vi "BuildPacketJ1939.vi"(7 "Priority":u8=6 format="%x", 9 "SA":u8, 10 "Data":u8[](array[numeric]), 11 "TxID":u8) -> (2 "MsgTX 2":T1)   [LabVIEW 2017]
panel:
  out "PGN":u16
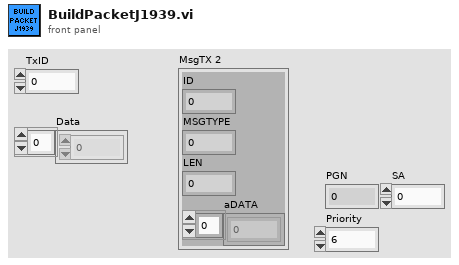
[diagram p1: front panel]
types:
  T1 = cluster{"ID":u32, "MSGTYPE":u8, "LEN":u8, "aDATA":u8[]}
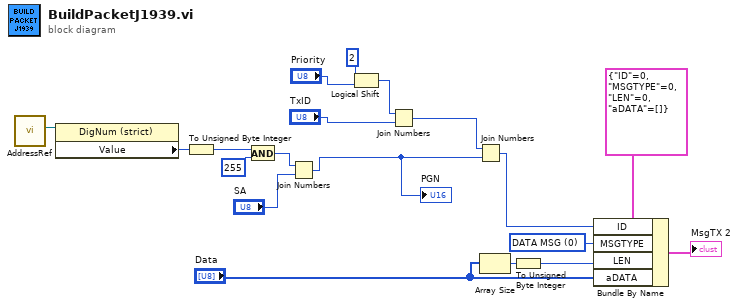
[diagram p0: block diagram]
diagram:
  w19 = u8 0 items=["STATUS"=128, "EXTENDED"=2, "RTR"=1, "DATA MSG"=0] ("MSGTYPE")
  n1 = call "AddressRef.vi"() -> ("add_type out"=w14:refnum<vi>)  [unwired: 9 in, 2 out]
  n2 = property class="DigNum (strict)"(reference=w14) -> ("Value"=w7:u16)  [unwired: 1 in, 2 out]
  n3 = To Unsigned Byte Integer(number=w7) -> (unsigned 8bit integer=w4:u8)
  n4 = And(x=w4, y=u8 255) -> (x .and. y?=w3:u8)
  n5 = Join Numbers(hi=w3, lo="SA") -> ((hi.lo)=w5:u16)
  "PGN" <- w5
  n6 = Logical Shift(y=i16 2, x="Priority") -> (x << y=w11:u8)
  n7 = Join Numbers(hi=w11, lo="TxID") -> ((hi.lo)=w8:u16)
  n8 = Join Numbers(hi=w8, lo=w5) -> ((hi.lo)=w13:u32)
  n9 = Array Size(array="Data") -> (size(s)=w15:i32)
  n10 = To Unsigned Byte Integer(number=w15) -> (unsigned 8bit integer=w18:u8)
  n11 = Bundle By Name(cluster=T1 {"ID"=0, "MSGTYPE"=0, "LEN"=0, "aDATA"=[]} ("MsgTX 2"), "ID"=w13, "MSGTYPE"=w19, "LEN"=w18, "aDATA"="Data") -> (→"MsgTX 2":T1)
